vi "Open HTML Report in Browser (String).vi"(0 "URL":string, 11 "error in (no error)":errorcluster) -> (4 "URL out":string, 15 "error out":errorcluster)   [LabVIEW 2017, in "NI_ReportGenerationCore.lvlib"]
doc: "Displays an HTML report in the default Web browser. Wire data to the <B>report in</B> input to determine the polymorphic instance to use or manually select the instance. You cannot use this VI with standard reports."
uses:
  <vilib>/Utility/NIReport.llb/NI_ReportGenerationCore.lvlib
  <vilib>/Platform/browser.llb/Open URL in Default Browser (string).vi
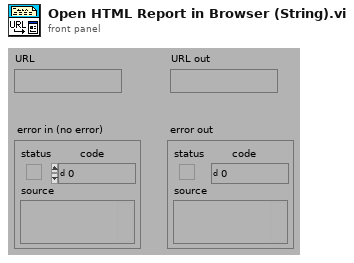
[diagram p1: front panel]
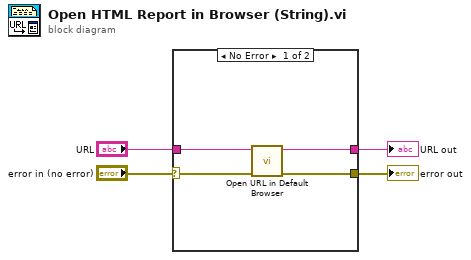
[diagram p0: block diagram]
diagram:
  n1 = case shown="No Error" "error in (no error)" {
    selector: "error in (no error)" -> [w7 w10]
    tunnel: [w8 w10] -> w3
    tunnel: "URL" -> [w6 w9]
    tunnel: [w5 w9] -> w1
    frame No Error {
      n2 = call-poly <vilib>:"Open URL in Default Browser.vi"("error in (no error)"=w7, "URL"=w6) -> ("error out"=w8:errorcluster, "URL out"=w5:string)  [unwired: 4 in]
    }
    frame Error {
    }
  }
  "error out" <- w3
  "URL out" <- w1
